vi "log_downloader.vi"() -> ()   [LabVIEW 2022 SP3]
uses:
  LabSSH Library/SSH Library/Connection Info..cluster.ctl
  <vilib>/Utility/miscctls.llb/LVPointTypeDef.ctl
  LabSSH Library/SSH Library/LabSSH.lvlib
panel:
  in  "cmd Time (s)":dbl=3.0 format="%#_13g"
  in  "remote path":string(combo)
  in  "fileTree":string(tree)
  in  "explore":bool
  in  "address":string(combo)="192.168.1.200"
  in  "sftp_get_log":bool
  in  "ssh generat log":bool
  in  "remoteFilePath":string
  in  "cmd Box 2":string(combo)="journalctl -u zipx.s.service -n 10000 "
  out "cmd string":string
  in  "Port":u16(ring)=22 items=["22"=22, "10060"=10060, "10070"=10070, "10080"=10080, "10090"=10090]
  in  "user":string(combo)="tvt"
  in  "Local folder":path
  out "exit":bool
  out "ip":string
  in  "stop":bool
  # "journalctl -u zipx.s.service -n 10000 |grep error"
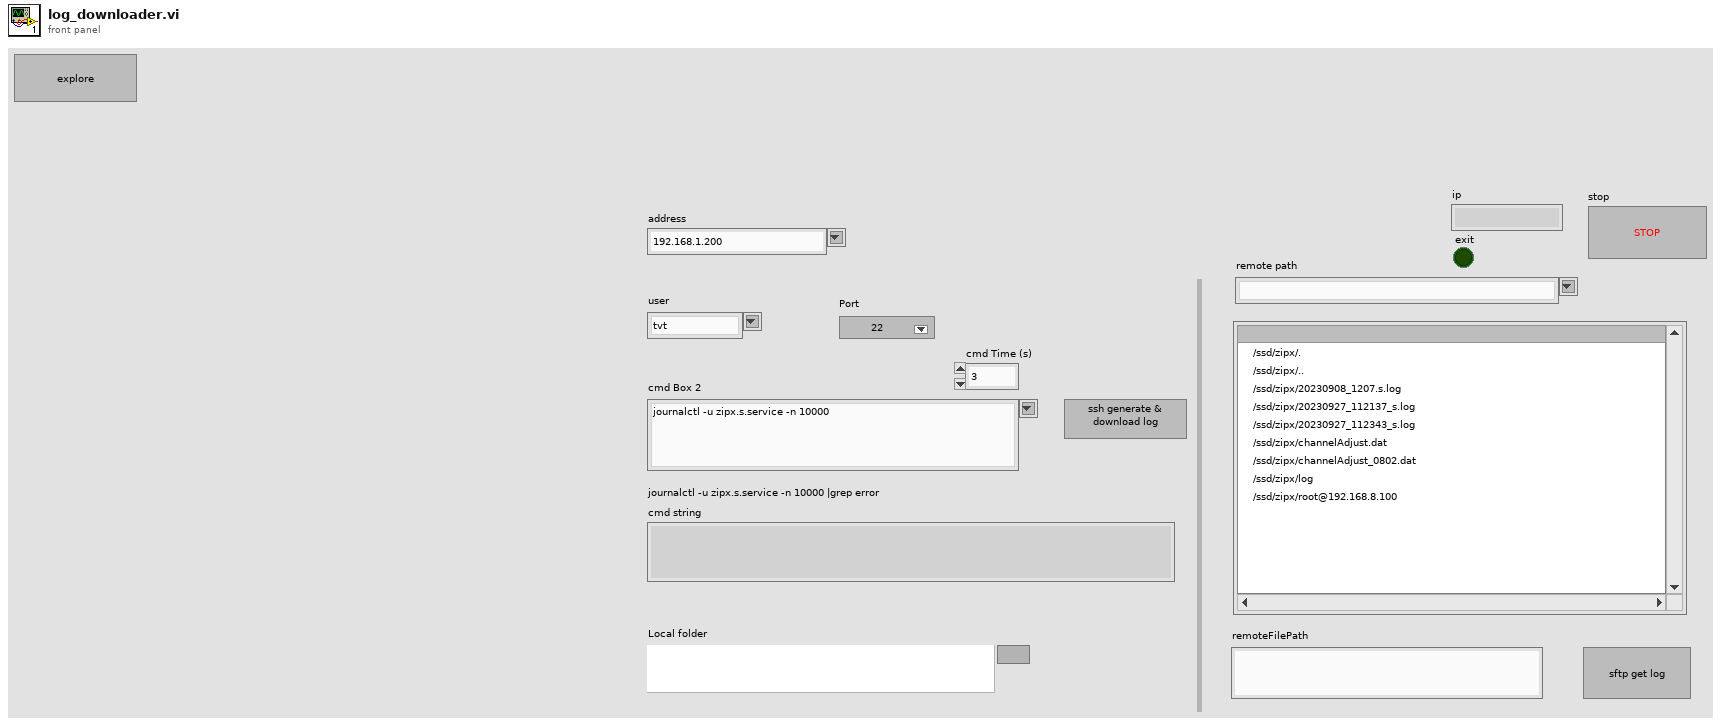
[diagram p1: front panel]
types:
  T1 = enum32{"Invalid", "Standard", "Closed", "Hidden", "Minimized", "Maximized"}
  T2 = typedef "LabSSH.lvlib/Connection Info..cluster.ctl" = cluster{"Remote":string, "Username":string, "Port (22)":i32}
  T3 = typedef "LVPointTypeDef.ctl" = cluster{"Horizontal":i16, "Vertical":i16}
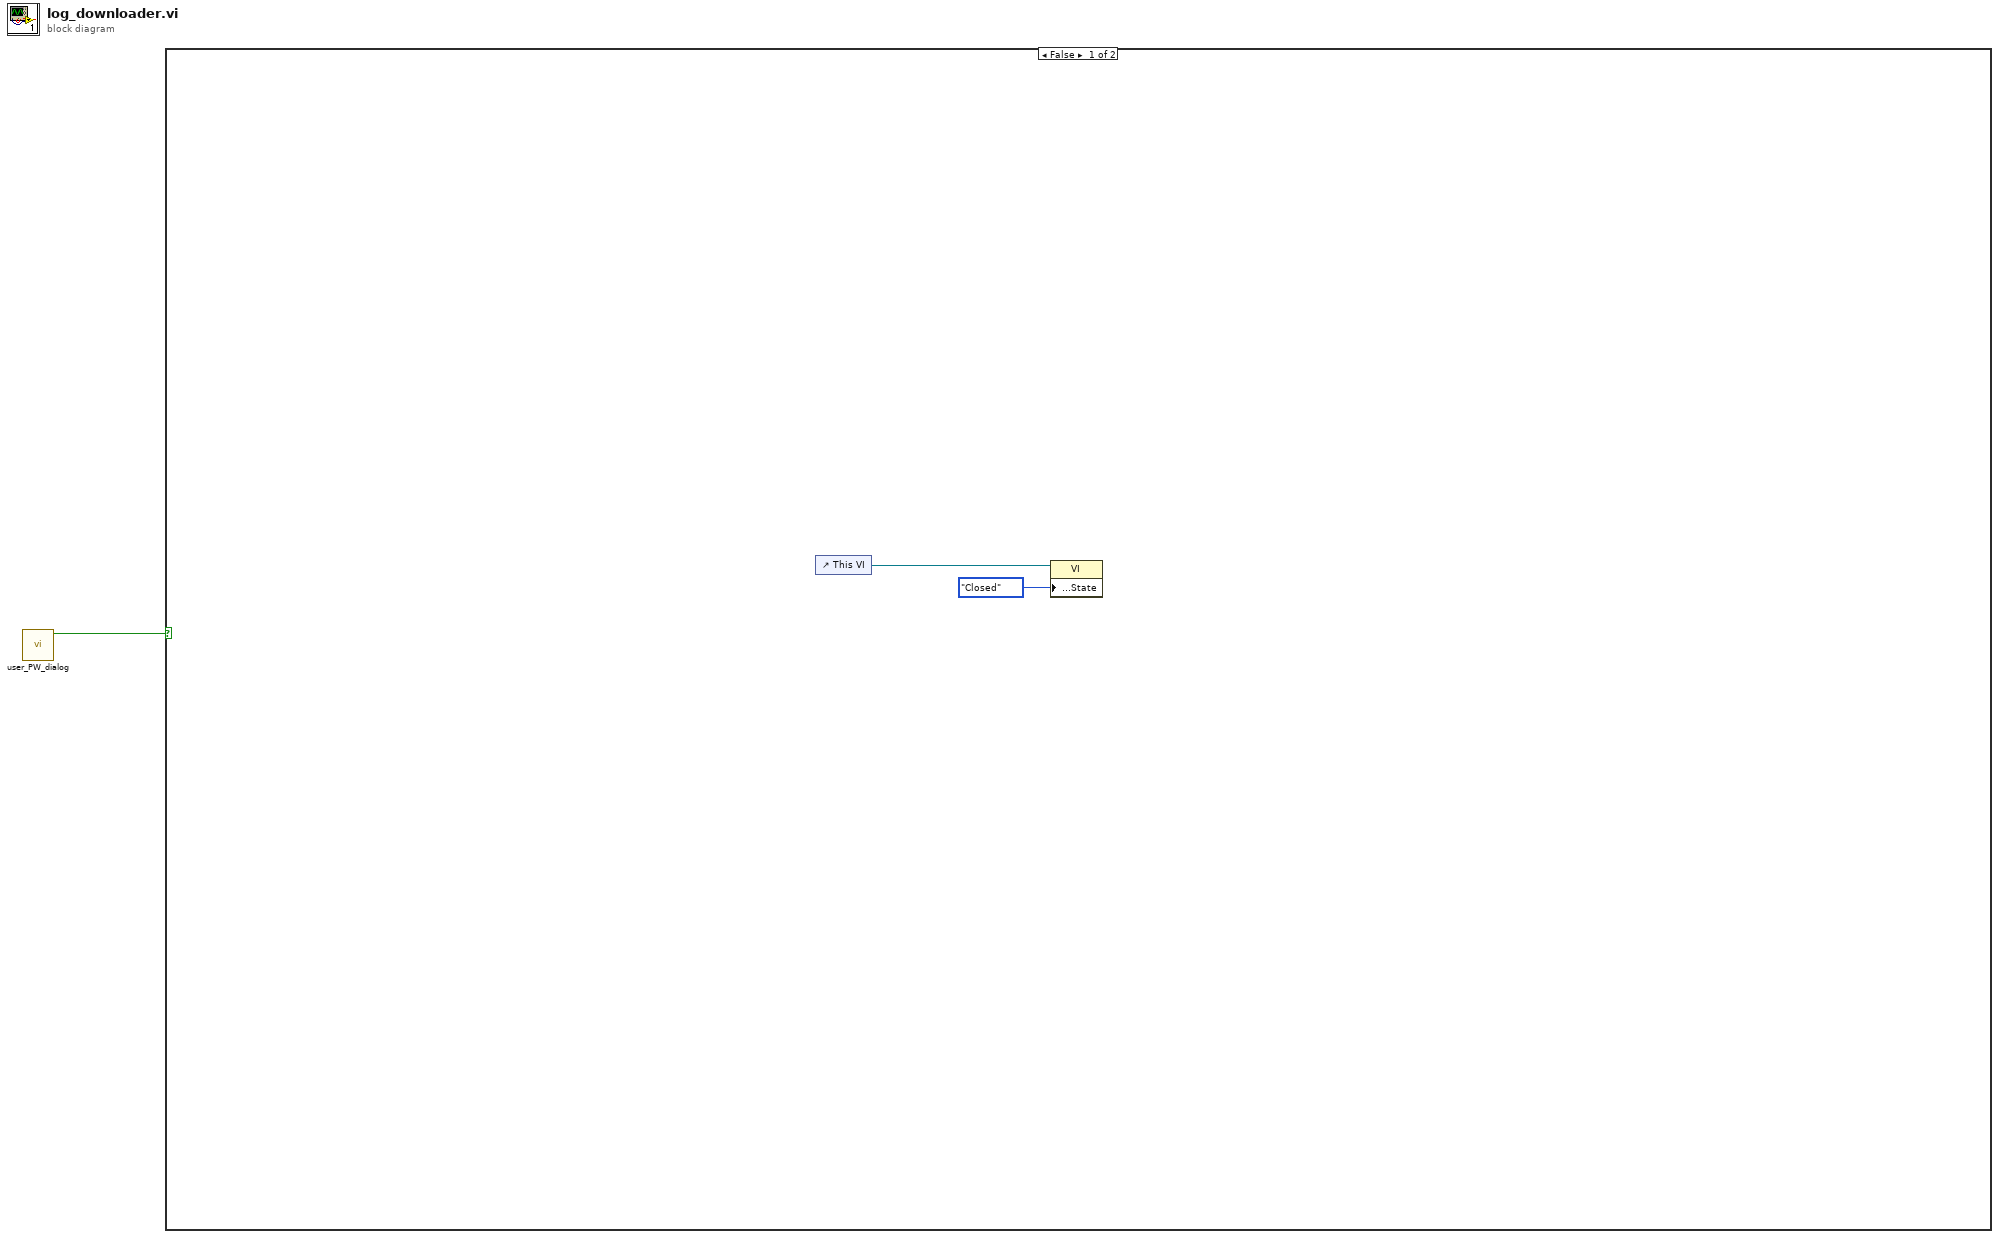
[diagram p0: block diagram]
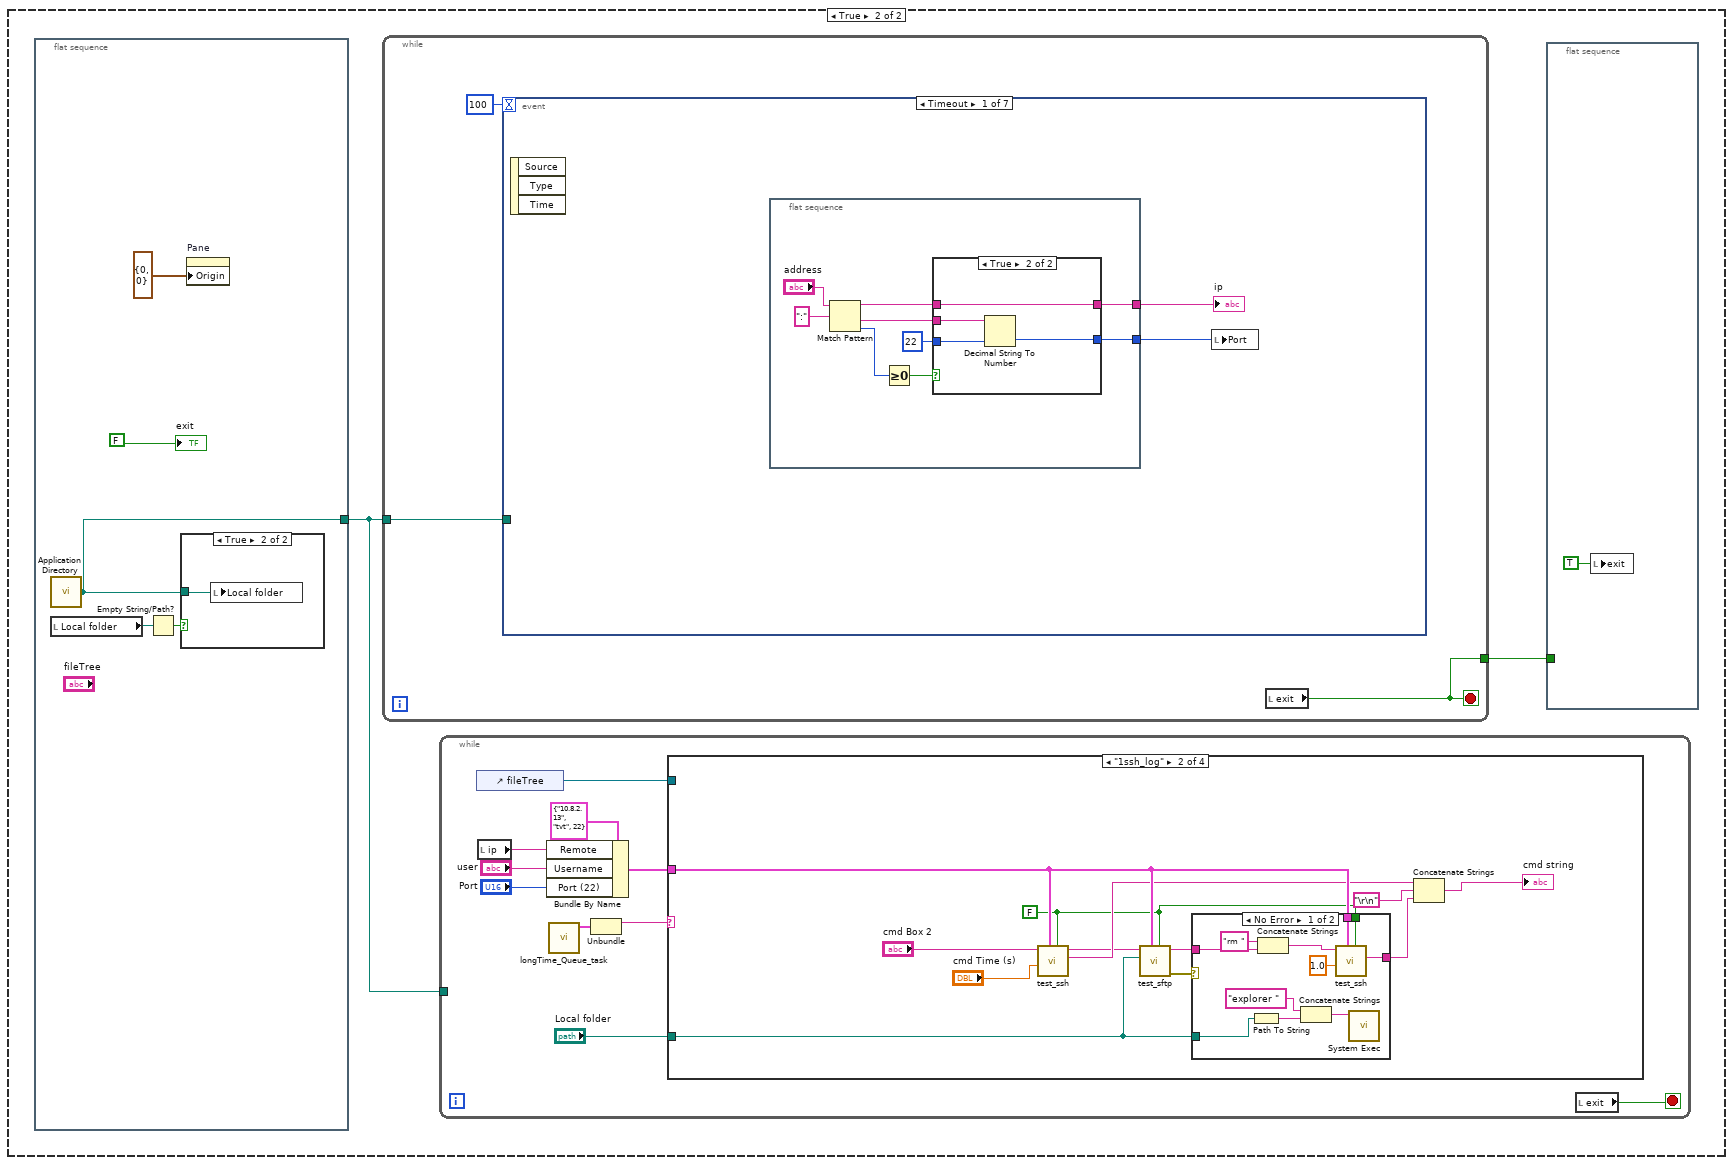
[diagram p2: hidden frame]
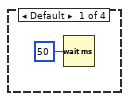
[diagram p3: hidden frame]
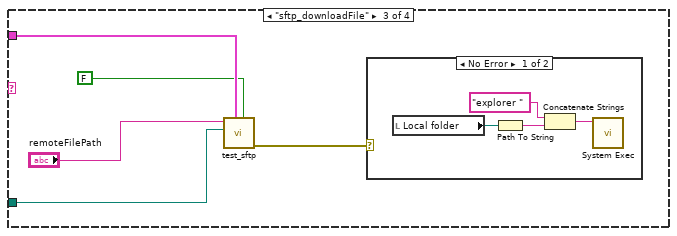
[diagram p5: hidden frame]
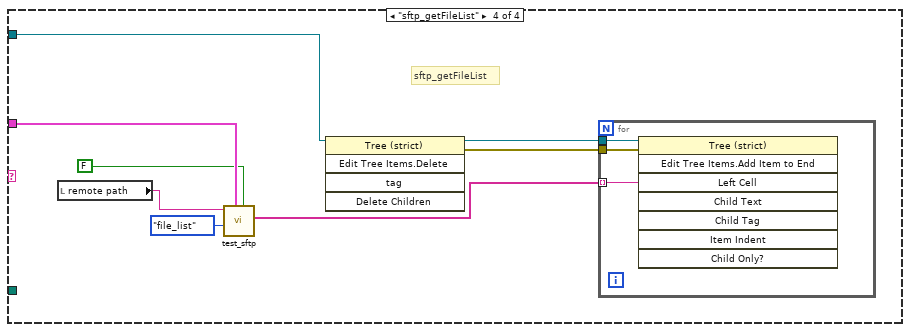
[diagram p7: hidden frame]
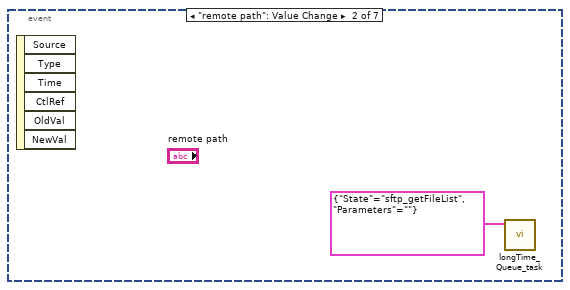
[diagram p10: hidden frame]
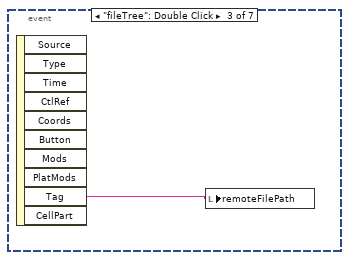
[diagram p11: hidden frame]
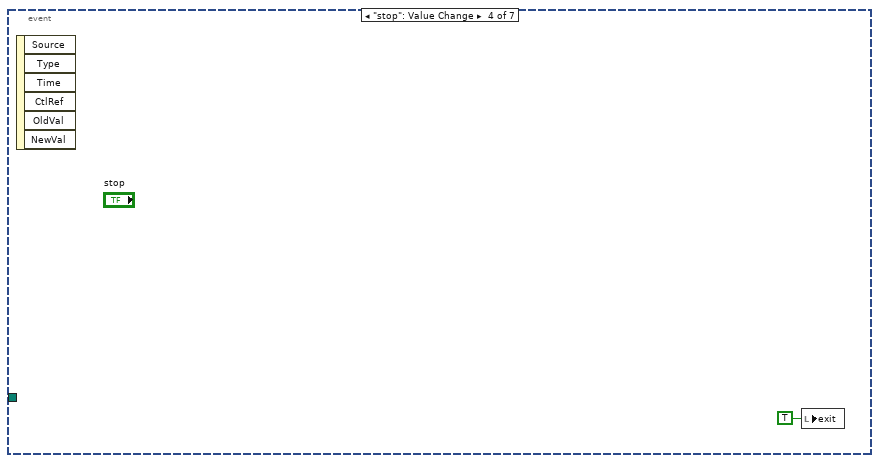
[diagram p12: hidden frame]
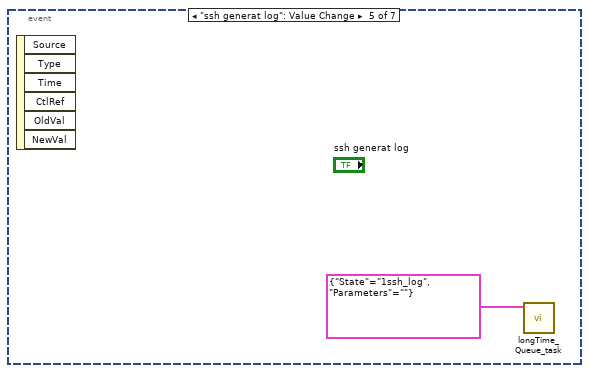
[diagram p13: hidden frame]
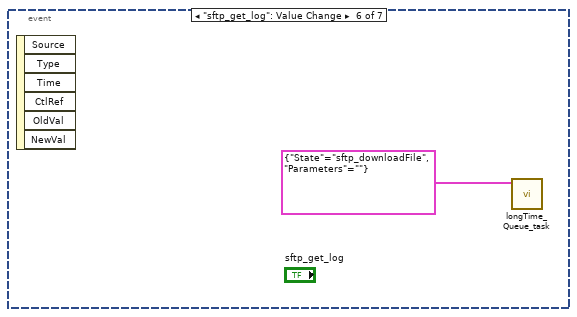
[diagram p14: hidden frame]
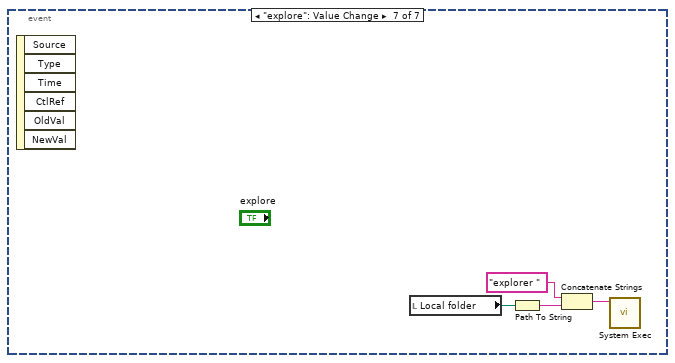
[diagram p15: hidden frame]
diagram:
  n1 = call "user_PW_dialog.vi"() -> ("result"=w1:bool)  [unwired: 11 in]
  n2 = case shown="False" w1 {
    frame False {
      n3 = control-ref of="This VI"() -> (w2:refnum<vi>)
      n4 = property class="VI"(reference=w2, "Front Panel Window:State"=T1."Closed") -> ()  [unwired: 1 in, 2 out]
    }
    frame True {
      n5 = flat-sequence {
        tunnel: [w62] -> w5
        frame #0 {
          n6 = call <vilib>:"Application Directory.vi"() -> ("Application Directory"=w62:path)
          n7 = local read "Local folder"() -> (w64:path)
          n8 = Empty String/Path?(string/path=w64) -> (empty?=w63:bool)
          n9 = case shown="True" w63 {
            tunnel: w62 -> [_ w65]
            frame False {
            }
            frame True {
              n10 = local write "Local folder"(w65) -> ()
            }
          }
          n11 = property on="Pane" class="Pane"("Origin"=T3 {"Horizontal"=0, "Vertical"=0}) -> ()  [unwired: 2 in, 2 out]
          "exit" <- FALSE ("stop")
        }
      }
      n12 = while {
        tunnel: w5 -> [w67]
        tunnel: [w66] -> w4
        stop <- w66 stop-if-true
        n13 = event shown="[0] Timeout" {
          selector: _ -> [_ _ _ _ _ _ _]
          dyn-events: _ -> [_ _ _ _ _ _ _]
          timeout: 100 -> [_ _ _ _ _ _ _]
          tunnel: w67 -> [_ _ _ _ _ _ _]
          event Timeout {
            n14 = event-data() -> ()  [unwired: 1 in, 3 out]
            n15 = flat-sequence {
              tunnel: [w73] -> w70
              tunnel: [w72] -> w69
              frame #0 {
                n16 = Match Pattern(string="address", regular expression=":") -> (before substring=w77:string, after substring=w76:string, offset past match=w79:i32)  [unwired: 1 in, 1 out]
                n17 = Greater Or Equal To 0?(x=w79) -> (x >= 0?=w78:bool)
                n18 = case shown="True" w78 {
                  tunnel: w77 -> [w80 w83]
                  tunnel: w76 -> [_ w85]
                  tunnel: u16 22 ("remote port or service name") -> [w81 w84]
                  tunnel: [w80 w83] -> w73
                  tunnel: [w81 w82] -> w72
                  frame False {
                  }
                  frame True {
                    n19 = Decimal String To Number(string=w85, default (0L)=w84) -> (number=w82:u16)  [unwired: 1 in, 1 out]
                  }
                }
              }
            }
            n20 = local write "Port"(w69) -> ()
            "ip" <- w70
          }
          event "remote path": Value Change {
            n21 = event-data() -> ()  [unwired: 1 in, 6 out]
            n22 = call "longTime_Queue_task.vi"("taskInput"=cluster{"State":string, "Parameters":string} {"State"="sftp_getFileList", "Parameters"=""}) -> ()  [unwired: 9 in, 2 out]
          }
          event "fileTree": Double Click {
            n23 = event-data() -> ("Tag"=w87:string)  [unwired: 1 in, 9 out]
            n24 = local write "remoteFilePath"(w87) -> ()
          }
          event "stop": Value Change {
            n25 = event-data() -> ()  [unwired: 1 in, 6 out]
            n26 = local write "exit"(TRUE ("exit")) -> ()
          }
          event "ssh generat log": Value Change {
            n27 = event-data() -> ()  [unwired: 1 in, 6 out]
            n28 = call "longTime_Queue_task.vi"("taskInput"=cluster{"State":string, "Parameters":string} {"State"="1ssh_log", "Parameters"=""}) -> ()  [unwired: 9 in, 2 out]
          }
          event "sftp_get_log": Value Change {
            n29 = event-data() -> ()  [unwired: 1 in, 6 out]
            n30 = call "longTime_Queue_task.vi"("taskInput"=cluster{"State":string, "Parameters":string} {"State"="sftp_downloadFile", "Parameters"=""}) -> ()  [unwired: 9 in, 2 out]
          }
          event "explore": Value Change {
            n31 = event-data() -> ()  [unwired: 1 in, 6 out]
            n32 = local read "Local folder"() -> (w92:path)
            n33 = Path To String(path=w92) -> (string=w93:string)
            n34 = Concatenate Strings("explorer " ("string"), w93) -> (w94:string)
            n35 = call <vilib>:"System Exec.vi"("command line"=w94) -> ()  [unwired: 7 in, 4 out]
          }
        }
        n36 = local read "exit"() -> (w66:bool)
      }
      n37 = while {
        tunnel: w5 -> [_]
        stop <- w14 stop-if-true
        n38 = control-ref of="fileTree"() -> (w8:refnum<vi>)
        n39 = local read "ip"() -> (w11:string)
        n40 = Bundle By Name(cluster=T2 {"Remote"="10.8.2.13", "Username"="tvt", "Port (22)"=22} ("Connection Info."), "Remote"=w11, "Username"="user", "Port (22)"="Port") -> (w9:T2)
        n41 = call "longTime_Queue_task.vi"() -> ("taskOut"=w16:cluster{"State":string, "Parameters":string})  [unwired: 10 in, 1 out]
        n42 = Unbundle(w16) -> ("State"=w15:string)  [unwired: 1 out]
        n43 = case shown="\"1ssh_log\"" w15 {
          tunnel: w9 -> [_ w26 w44 w56]
          tunnel: w8 -> [_ _ _ w50]
          tunnel: "Local folder" -> [_ w18 w40 _]
          frame Default {
            n44 = Wait (ms)(milliseconds to wait=u32 50) -> ()  [unwired: 1 out]
          }
          frame "1ssh_log" {
            w23 = FALSE ("Close?")
            n45 = call "test_ssh.vi"("Close?"=w23, "Connection Info."=w26, "Delay Time (s)"="cmd Time (s)", "cmd Box"="cmd Box 2") -> ("cmd string"=w25:string, "remote log path"=w24:string)  [unwired: 5 in, 1 out]
            n46 = call "test_sftp.vi"("Close"=w23, "Connection Info."=w26, "Local folder"=w18, "Remote File Path"=w24) -> ("error out"=w20:errorcluster)  [unwired: 6 in, 1 out]
            n47 = case shown="No Error" w20 {
              tunnel: w24 -> [w38 _]
              tunnel: w26 -> [w36 _]
              tunnel: w23 -> [w35 _]
              tunnel: [w34 _] -> w22
              tunnel: w18 -> [w29 _]
              frame No Error {
                n48 = Path To String(path=w29) -> (string=w31:string)
                n49 = Concatenate Strings("rm " ("string"), w38) -> (w37:string)
                n50 = Concatenate Strings("explorer " ("string"), w31) -> (w32:string)
                n51 = call "test_ssh.vi"("Close?"=w35, "Connection Info."=w36, "Delay Time (s)"=1.0, "cmd Box"=w37) -> ("cmd string"=w34:string)  [unwired: 5 in, 2 out]
                n52 = call <vilib>:"System Exec.vi"("command line"=w32) -> ()  [unwired: 7 in, 4 out]
              }
              frame Error {
              }
            }
            n53 = Concatenate Strings(w25, "\r\n", w22) -> (→"cmd string":string)
          }
          frame "sftp_downloadFile" {
            n54 = call "test_sftp.vi"("Close"=FALSE ("Close?"), "Connection Info."=w44, "Local folder"=w40, "Remote File Path"="remoteFilePath") -> ("error out"=w42:errorcluster)  [unwired: 6 in, 1 out]
            n55 = case shown="No Error" w42 {
              frame No Error {
                n56 = local read "Local folder"() -> (w47:path)
                n57 = Path To String(path=w47) -> (string=w46:string)
                n58 = Concatenate Strings("explorer " ("string"), w46) -> (w45:string)
                n59 = call <vilib>:"System Exec.vi"("command line"=w45) -> ()  [unwired: 7 in, 4 out]
              }
              frame Error {
              }
            }
          }
          frame "sftp_getFileList" {
            # "sftp_getFileList"
            n60 = local read "remote path"() -> (w49:string)
            n61 = call "test_sftp.vi"("Close"=FALSE ("Close?"), "Connection Info."=w56, "Operation"=enum16{"DownLoad", "file_list"}."file_list", "Remote File Path"=w49) -> ("folder&file List"=w54:string[])  [unwired: 6 in, 1 out]
            n62 = invoke on="Invoke Node" class="Tree (strict)" method="Edit Tree Items.Delete"(reference=w50) -> (reference out=w53:refnum<vi>, error out=w52:errorcluster)  [unwired: 4 in, 3 out]
            n63 = for {
              tunnel: w53 -> [w59]
              tunnel: w52 -> [w58]
              tunnel: w54 -> [w57] mode=indexing
              n64 = invoke on="Invoke Node" class="Tree (strict)" method="Edit Tree Items.Add Item to End"(reference=w59, error in=w58, "Left Cell"=w57) -> ()  [unwired: 5 in, 8 out]
            }
          }
        }
        n65 = local read "exit"() -> (w14:bool)
      }
      n66 = flat-sequence {
        tunnel: w4 -> [_]
        frame #0 {
          n67 = local write "exit"(TRUE ("stop")) -> ()
        }
      }
    }
  }
